vi "COMMotor.vi"(3 "Target [mm]":dbl format="%.3p", 4 "ustep":u16(ring)=2 items=["full"=1, "1/2"=2, "1/4"=4, "1/8"=8, "1/16"=16], 5 "axis":u16(ring) items=["X", "Y", "Z"], 6 "VISA in":refnum<visa-resource-name>="COM1") -> (0 "Moving":bool, 1 "Position [mm]":dbl format="%.3p", 2 "VISA out":refnum<visa-resource-name>="COM1")   [LabVIEW 2022 SP3]
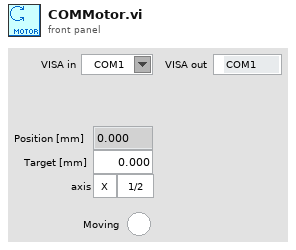
[diagram p1: front panel]
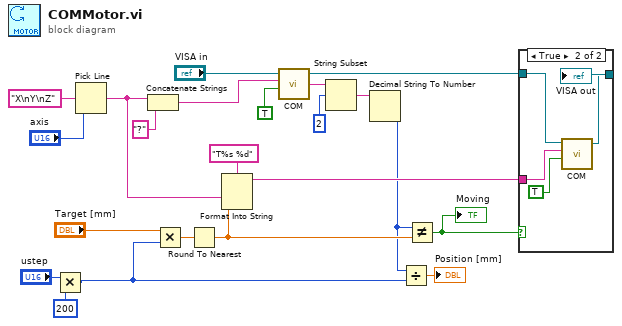
[diagram p0: block diagram]
diagram:
  n1 = Multiply(x="ustep", y=u16 200) -> (x*y=w1:u16)
  n2 = Pick Line(multi-line string="X\nY\nZ", line index="axis") -> (output string=w18:string)  [unwired: 1 in]
  n3 = Concatenate Strings(w18, "?" ("string")) -> (w16:string)
  n4 = Multiply(x="Target [mm]", y=w1) -> (x*y=w4:dbl)
  n5 = Round To Nearest(number=w4) -> (nearest integer value=w10:dbl)
  n6 = Format Into String(format string="T%s %d", w18, w10) -> (resulting string=w8:string)  [unwired: 2 in, 1 out]
  n7 = call "COM.vi"("Write?"=TRUE, "command"=w16, "VISA in"="VISA in") -> ("reply"=w13:string, "VISA out"=w9:refnum<visa-resource-name>)  [unwired: 1 in, 1 out]
  n8 = String Subset(string=w13, offset (0)=2) -> (substring=w11:string)  [unwired: 1 in]
  n9 = Decimal String To Number(string=w11) -> (number=w5:i32)  [unwired: 2 in, 1 out]
  n10 = Divide(x=w5, y=w1) -> (x/y=→"Position [mm]":dbl)
  n11 = Not Equal?(x=w5, y=w10) -> (x != y?=w6:bool)
  "Moving" <- w6
  n12 = case shown="True" w6 {
    tunnel: w9 -> [w24 w28]
    tunnel: w8 -> [_ w27]
    tunnel: [w24 w25] -> w7
    frame False {
    }
    frame True {
      n13 = call "COM.vi"("Write?"=TRUE, "command"=w27, "VISA in"=w28) -> ("VISA out"=w25:refnum<visa-resource-name>)  [unwired: 1 in, 2 out]
    }
  }
  "VISA out" <- w7
